vi "Host main_old.vi"() -> ()   [LabVIEW 2013]
uses:
  <vilib>/rvi/interface/nirviReadWriteControl/nirviReadWriteControl.xnode
  <vilib>/rvi/errors/niLvFpgaAdjustHostInterfaceError.vi
  <vilib>/rvi/interface/nirviCloseFPGA/nirviCloseFPGA.xnode
  FPGA/DataMode.ctl
  <vilib>/Utility/error.llb/Error Cluster From Error Code.vi
  <vilib>/rvi/interface/Simulation/niFpgaSimulationCallBeginRW.vi
  Host/Utilities/Ticker/Ticker.lvclass
  Host/Scope/controls/ScopeMode.ctl
  <vilib>/rvi/interface/nirviOpenFPGA/nirviOpenFPGA.xnode
  Host/Scope/P2P streaming/trigger_source.ctl
  Host/Config/FPGAref.ctl
  <userlib>/_OpenG.lib/file/file.llb/Valid Path - Traditional__ogtk.vi
  NiFpgaLv.dll
  FPGA Bitfiles/mixer_FPGATarget_FPGAmain_-FFnNgPrUUY.lvbitx
  <vilib>/FPGAPlugInAG/PXIe-7975R/niLvFpga_Open_PXIe-7975R.vi
  <vilib>/rvi/interface/common/dynamic/niFpgaDynamicAddResources.vi
  <vilib>/FPGAPlugInAG/Dynamic/niLvFpga_Close_Dynamic.vi
  <vilib>/userdefined/High Color/nirio_resource_hc.ctl
  <vilib>/Analysis/4window.llb/windowTd.ctl
  <vilib>/Analysis/NI_AALPro.lvlib
  Host/Scope/controls/power_spectrum_unit.ctl
panel:
  in  "Filter coefficients":path
  in  "Extra downsample":u16(ring) items=["None", "2", "3", "4", "5", "6", "7", "8", "9", "10", "11", "12", "13", "14", "15", "16"]
  in  "Enable extra FIR filter":bool
  in  "Ch1 Q":bool
  in  "Ch1 I":bool
  in  "Ch0 Q":bool
  in  "Ch0 I":bool
  in  "Ch1":bool
  in  "Ch0":bool
  out "stop 2":bool
  out "error out":errorcluster
  in  "Trigger":T1
  in  "Zoom freq X":bool
  in  "Zoom freq Y":bool
  in  "Zoom time Y":bool
  in  "Zoom time X":bool
  in  "Ch3":bool
  in  "Ch2":bool
  in  "Ch3 Q":bool
  in  "Ch3 I":bool
  in  "Ch2 Q":bool
  in  "Ch2 I":bool
  in  "input impedance":u32(ring) caption="Input Impedance" items=["1 mega ohm"=0, "50 ohms"=2]
  in  "SCOPE Resource":refnum<k15>="Dev1" caption="NI-Scope Resource"
  in  "Unit":T2
  in  "Window":T3=1 items=["Rectangle"=0, "Hanning"=1, "Hamming"=2, "Blackman-Harris"=3, "Exact Blackman"=4, "Blackman"=5, "Flat Top"=6, "4 Term B-Harris "=7, "7 Term B-Harris"=8, "Low Sidelobe"=9, "Blackman Nuttall"=11, "Triangle"=30, "Bartlett-Hanning"=31, "Bohman"=32, "Parzen"=33, "Welch"=34, "Kaiser"=60, "Dolph-Chebyshev"=61, "Gaussian"=62]
  in  "Samples per record":u32
  in  "Phase offset (deg)":dbl
  in  "Fequency [MHz]":dbl
  in  "Mode":T4
  in  "Mixer freq [MHz]":dbl
  in  "Ch1":bool
  in  "Ch0":bool
  out "freqdata":cluster{"f0":dbl, "df":dbl, "magnitude":dbl[]}[](graph)
  out "Timedata":i16[][](graph)
  in  "Rumode":bool
  in  "Singleshot":bool
  in  "Ch1 Q":bool
  in  "Ch1 I":bool
  in  "Ch0 Q":bool
  in  "Ch0 I":bool
  out "error IO":errorcluster
  in  "stop":bool
  in  "resource name":T5="RIO0"
  out "Clocking Option Configured?":bool
  out "Configured?":bool
  # "FPGA setup"
  # "Auto Zoom"
  # "Simulated data"
  # "5772"
  # "5160"
  # "Auto Zoom"
  # "FFT"
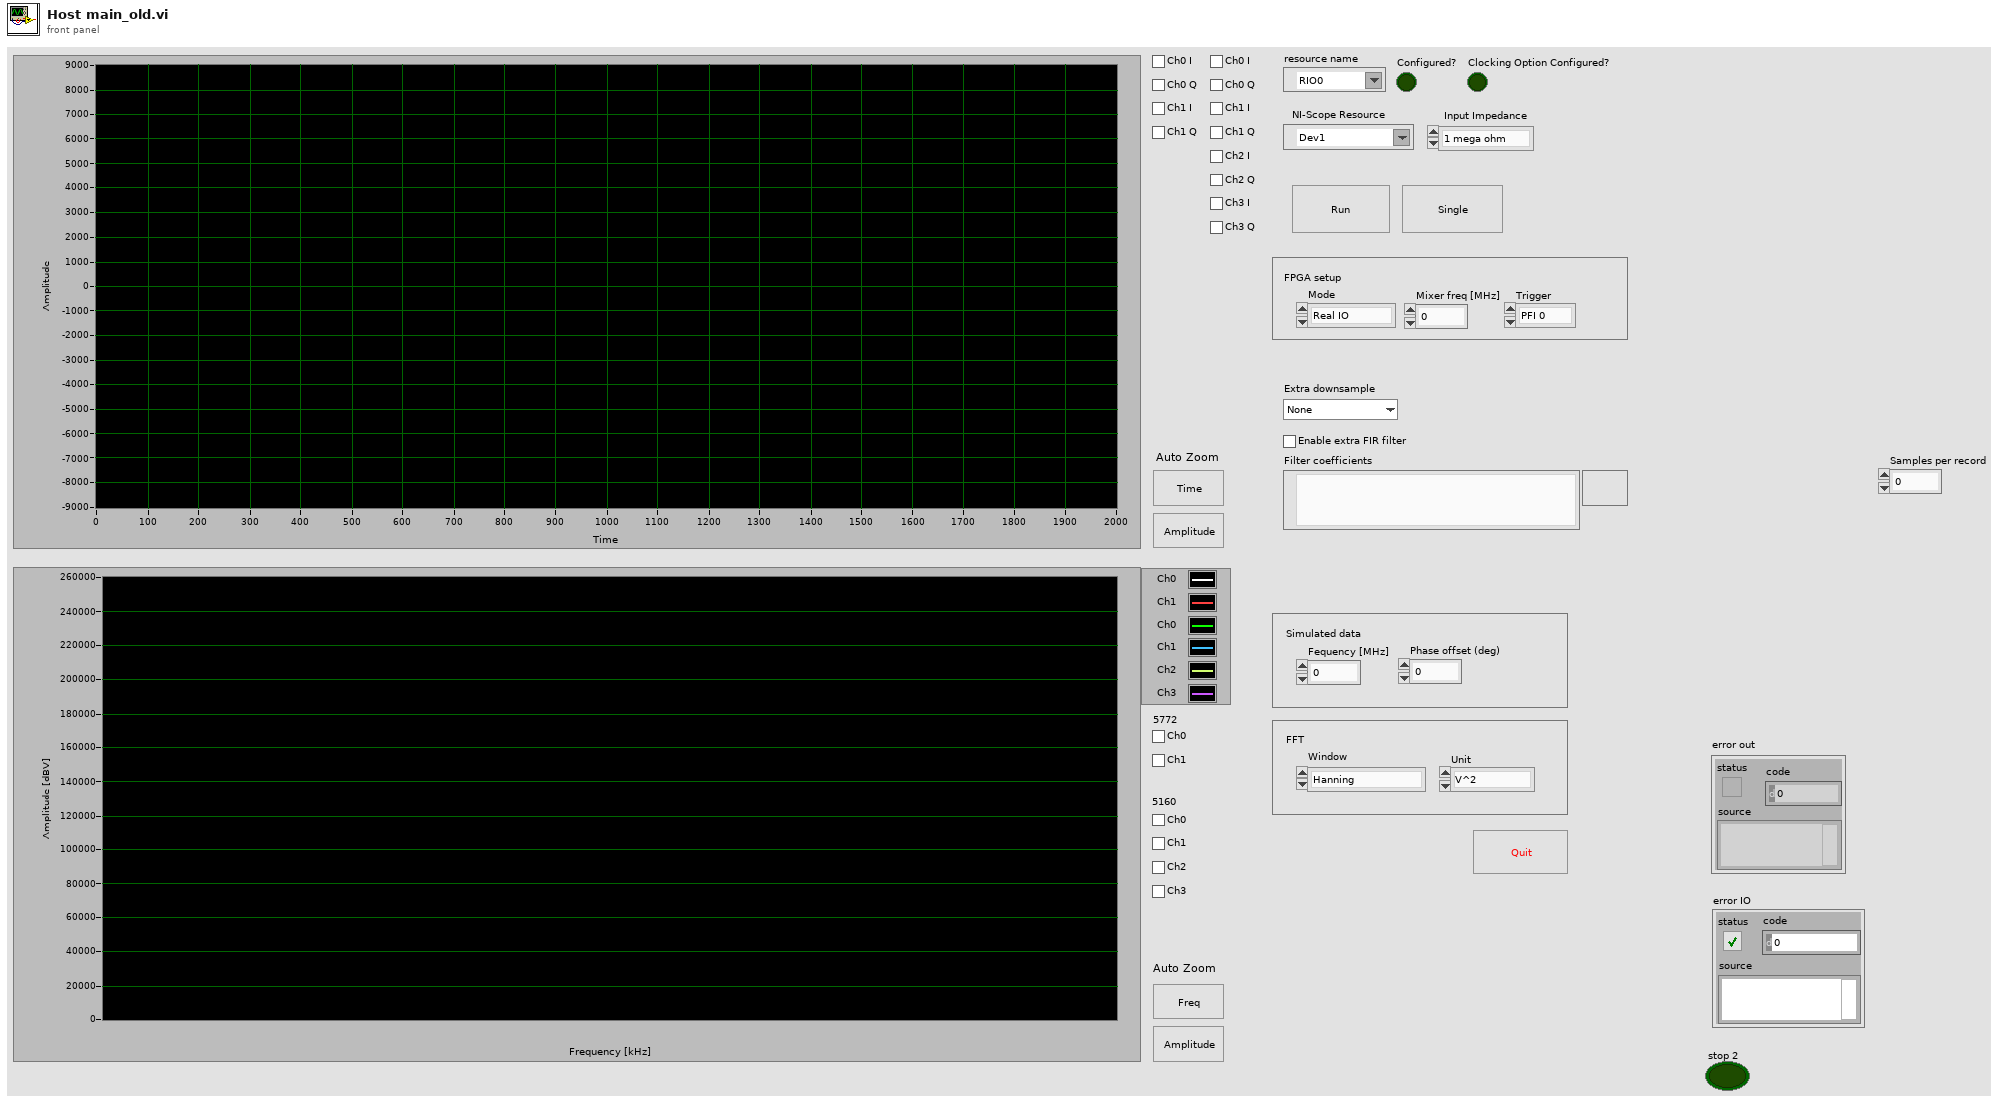
[diagram p1: front panel]
types:
  T1 = typedef "trigger_source.ctl" = enum16{"PFI 0", "PFI 1", "Software"}
  T2 = typedef "power_spectrum_unit.ctl" = enum16{"V^2", "V", "dBV"}
  T3 = typedef "NI_AALPro.lvlib/windowTd.ctl" = u32
  T4 = typedef "DataMode.ctl" = enum16{"Real IO", "Simulated"}
  T5 = typedef "nirio_resource_hc.ctl" = tag
  T6 = enum8{"Internal Clock PLL Off", "Internal Clock PLL On (REF IN)", "External Clock (CLK_IN)", "Internal Clock PLL On (IoModSyncClk)"}
  T7 = typedef "FPGAref.ctl" = refnum<k20>
  T8 = typedef "scope_params.ctl" = cluster{"scope mode":T9, "ticker":refnum<class "Ticker.lvclass">, "5160 samples per trigger":u32, "FPGA ref":T7, "P2P params":T10, "data mode":T4, "5782 samples per record":u32, "Chart length":i32}
  T9 = typedef "ScopeMode.ctl" = enum16{"Stopped", "Single", "Running", "Continuous"}
  T10 = typedef "P2P params.ctl" = cluster{"instrument handle":refnum<k15>, "stream session":refnum<k20>, "scale":cluster{"offset":dbl, "gain":dbl, "reserved 1":dbl, "reserved 2":dbl}, "actual sample rate":dbl, "Trigger":T1, "SCOPE Resource":refnum<k15>, "input impedance":u32}
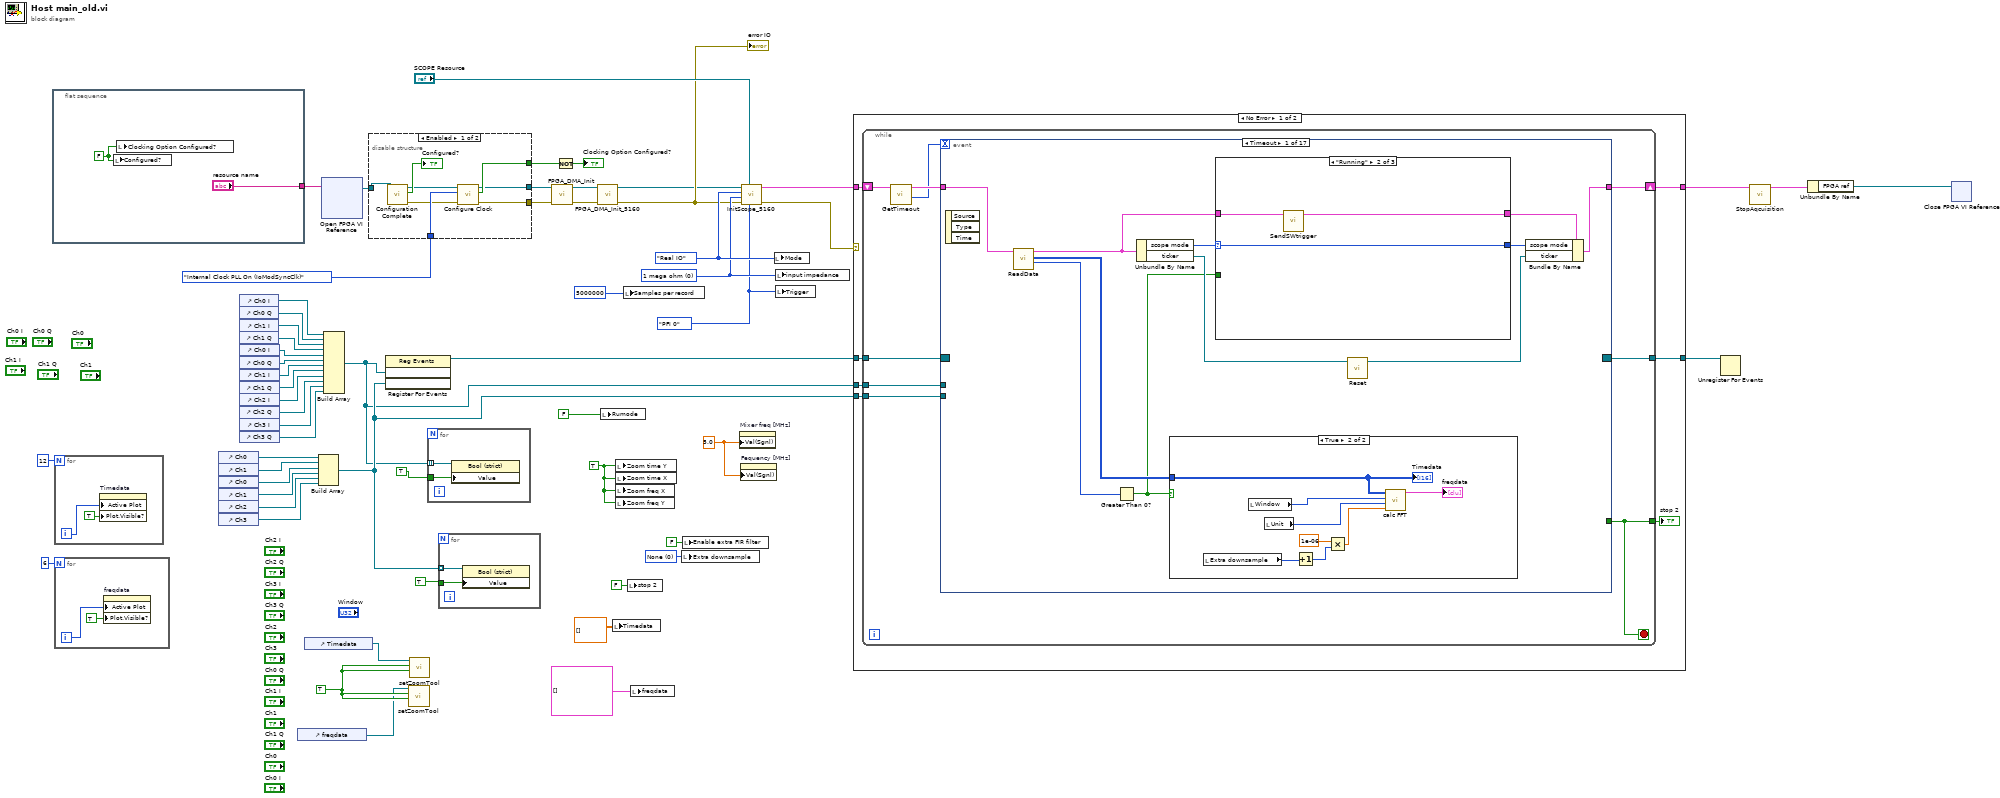
[diagram p0: block diagram]
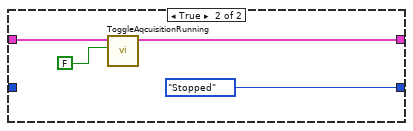
[diagram p6: hidden frame]
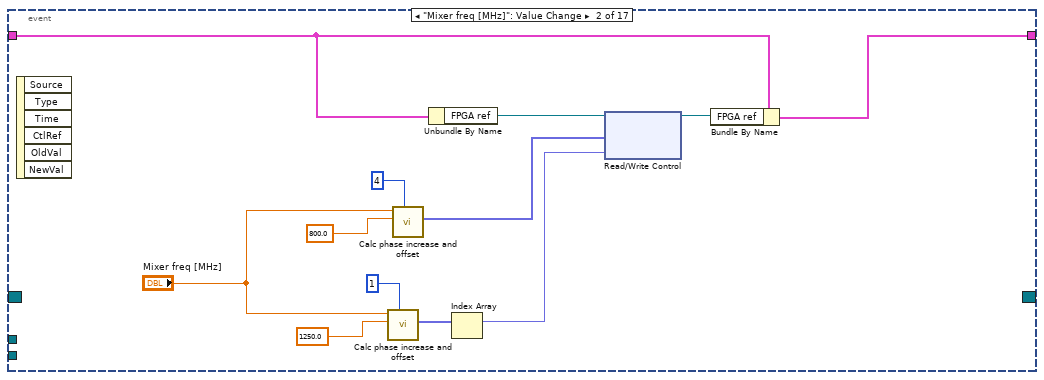
[diagram p7: hidden frame]
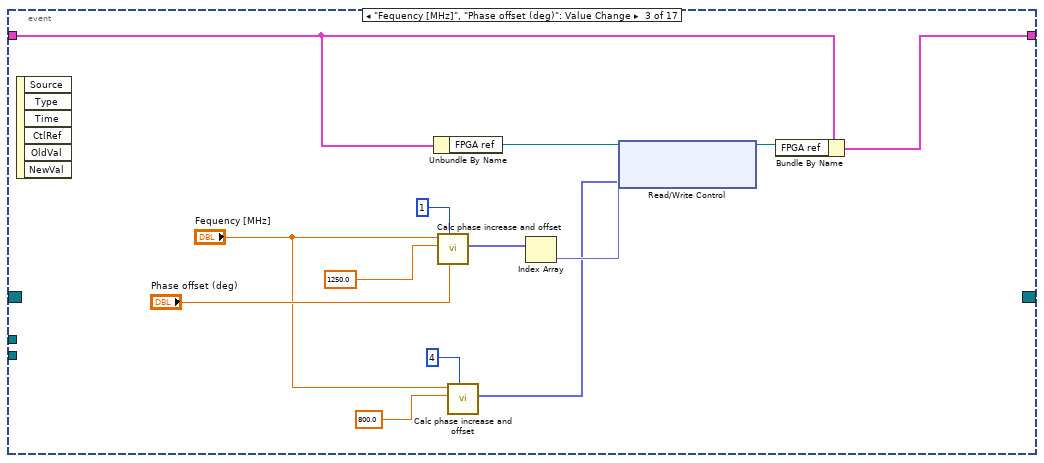
[diagram p8: hidden frame]
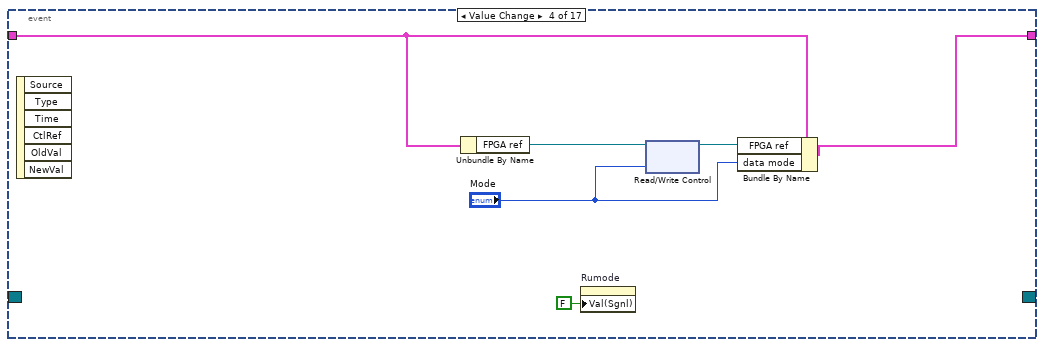
[diagram p9: hidden frame]
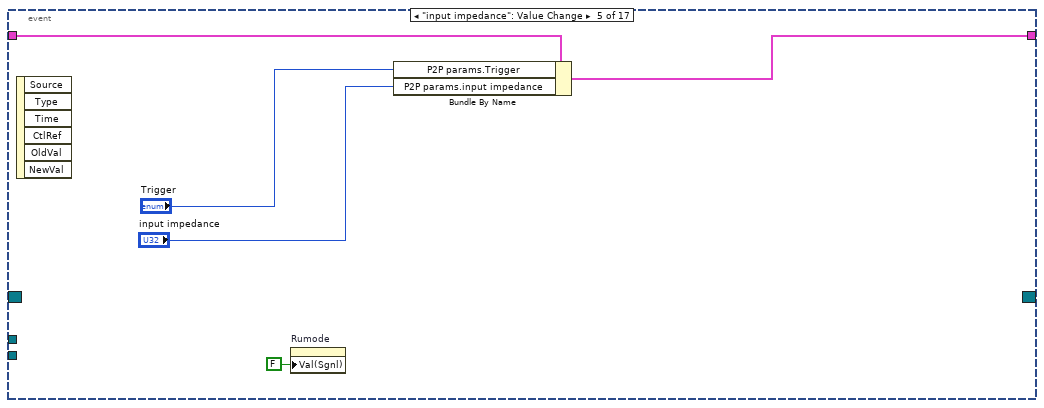
[diagram p10: hidden frame]
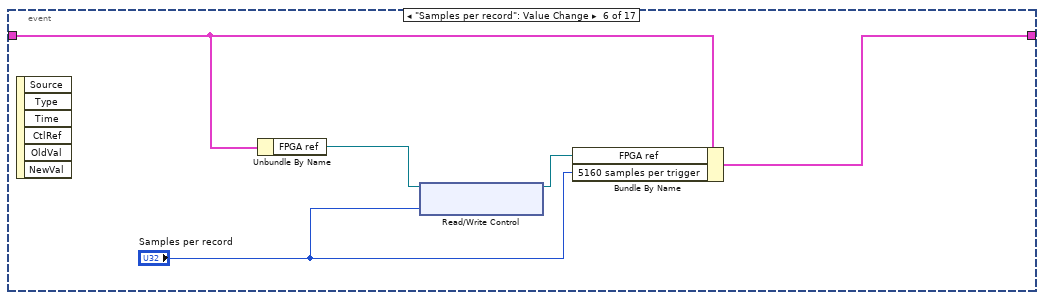
[diagram p11: hidden frame]
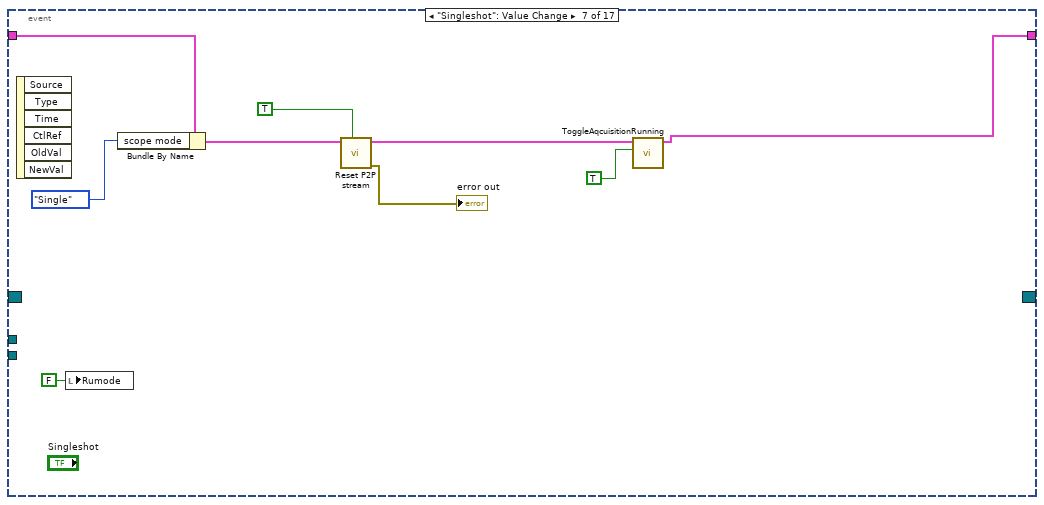
[diagram p12: hidden frame]
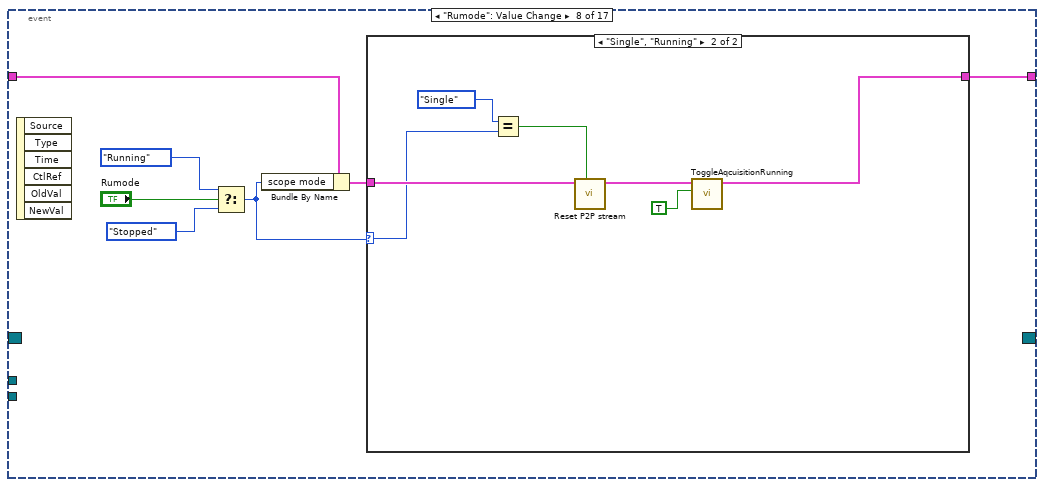
[diagram p13: hidden frame]
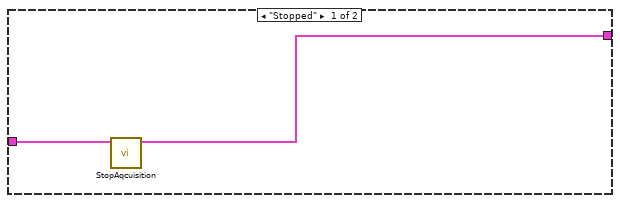
[diagram p14: hidden frame]
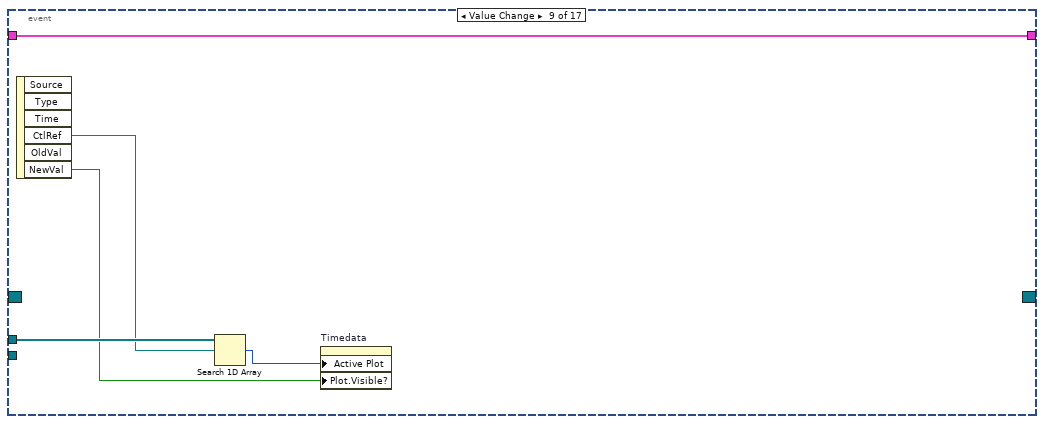
[diagram p15: hidden frame]
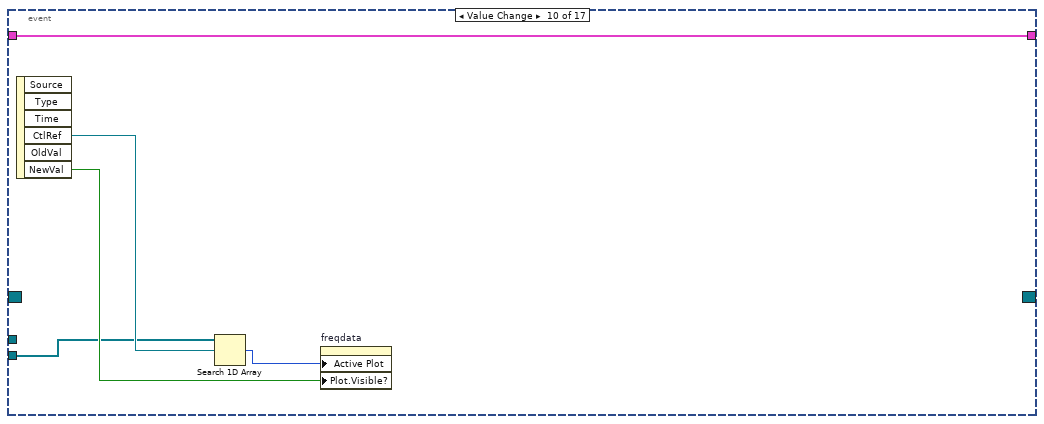
[diagram p16: hidden frame]
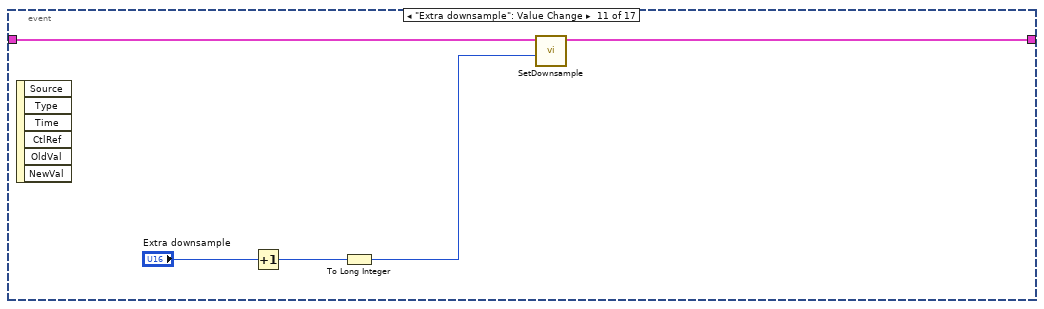
[diagram p17: hidden frame]
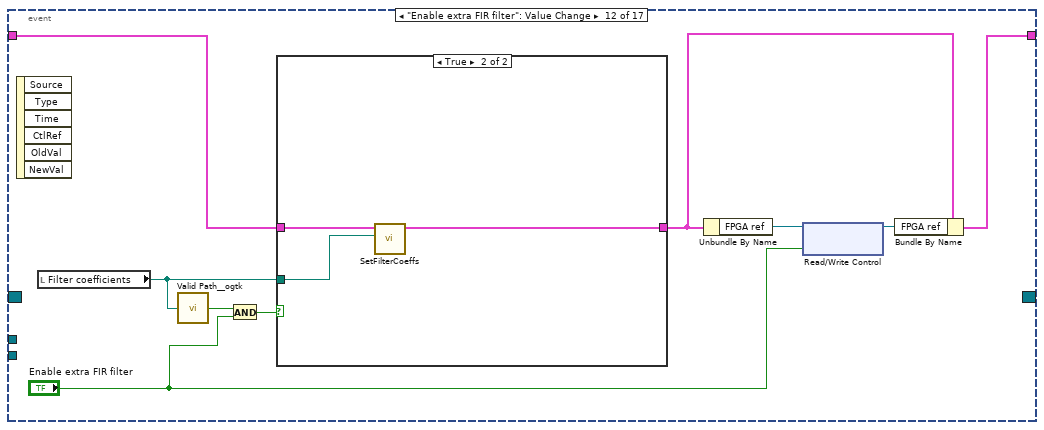
[diagram p18: hidden frame]
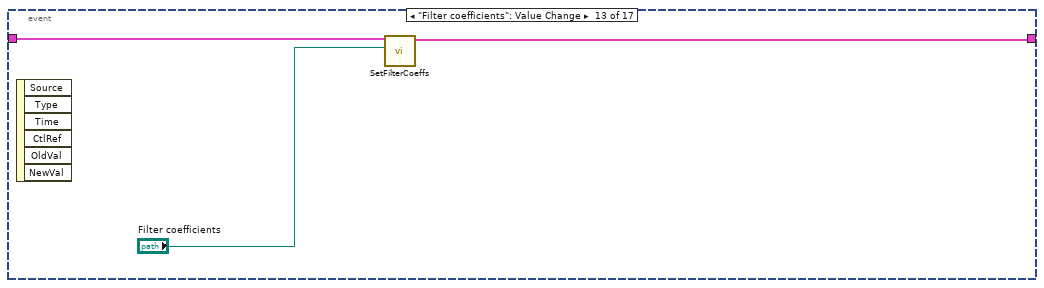
[diagram p20: hidden frame]
diagram:
  w3 = TRUE ("Zoom  X")
  w6 = u16 0 items=["None", "2", "3", "4", "5", "6", "7", "8", "9", "10", "11", "12", "13", "14", "15", "16"] ("Extra downsample")
  w20 = u32 0 items=["1 mega ohm"=0, "50 ohms"=2] ("input impedance")
  w16 = trigger_source."PFI 0" ("Trigger")
  w28 = TRUE ("Rumode")
  w21 = DataMode."Real IO" ("Mode")
  w54 = 5.0 ("Mixer requency [MHz]")
  n1 = flat-sequence {
    tunnel: ["resource name"] -> w29
    frame #0 {
      w59 = FALSE ("Trigger Acquisition")
      n2 = local write "Configured?"(w59) -> ()
      n3 = local write "Clocking Option Configured?"(w59) -> ()
    }
  }
  n4 = for {
    N: 12 -> [_]
    i -> [w62]
    n5 = property on="Timedata" class="WFGraph (strict)"("Active Plot"=w62, "Plot.Visible?"=TRUE ("Plot.Visible")) -> ()  [unwired: 2 in, 2 out]
  }
  n6 = for {
    N: 6 -> [_]
    i -> [w63]
    n7 = property on="freqdata" class="WFGraph (strict)"("Active Plot"=w63, "Plot.Visible?"=TRUE ("Plot.Visible")) -> ()  [unwired: 2 in, 2 out]
  }
  n8 = control-ref of="Ch0"() -> (w11:refnum<vi>)
  n9 = control-ref of="Ch1"() -> (w12:refnum<vi>)
  n10 = control-ref of="Ch0"() -> (w39:refnum<vi>)
  n11 = control-ref of="Ch1"() -> (w38:refnum<vi>)
  n12 = control-ref of="Ch2"() -> (w37:refnum<vi>)
  n13 = control-ref of="Ch3"() -> (w36:refnum<vi>)
  n14 = control-ref of="Ch0 I"() -> (w7:refnum<vi>)
  n15 = control-ref of="Ch0 Q"() -> (w8:refnum<vi>)
  n16 = control-ref of="Ch1 I"() -> (w9:refnum<vi>)
  n17 = control-ref of="Ch1 Q"() -> (w10:refnum<vi>)
  n18 = control-ref of="Ch0 I"() -> (w50:refnum<vi>)
  n19 = control-ref of="Ch0 Q"() -> (w49:refnum<vi>)
  n20 = control-ref of="Ch1 I"() -> (w48:refnum<vi>)
  n21 = control-ref of="Ch1 Q"() -> (w47:refnum<vi>)
  n22 = control-ref of="Ch2 I"() -> (w46:refnum<vi>)
  n23 = control-ref of="Ch2 Q"() -> (w45:refnum<vi>)
  n24 = control-ref of="Ch3 I"() -> (w44:refnum<vi>)
  n25 = control-ref of="Ch3 Q"() -> (w43:refnum<vi>)
  n26 = control-ref of="freqdata"() -> (w1:refnum<vi>)
  n27 = control-ref of="Timedata"() -> (w2:refnum<vi>)
  n28 = Build Array(w11, w12, w39, w38, w37, w36) -> (w34:refnum<vi>[])
  n29 = xnode "Open FPGA VI Reference"("resource name"=w29) -> ("FPGA VI Reference Out"=w26:refnum<k20>)  [unwired: 1 in, 1 out]
  n30 = Build Array(w7, w8, w9, w10, w50, w49, w48, w47, w46, w45, w44, w43) -> (w4:refnum<vi>[])
  n31 = disable-structure shown="Enabled" {
    disable-tunnel: [w71 _] -> w32
    disable-tunnel: T6."Internal Clock PLL On (IoModSyncClk)" ("Clock Source") -> [w70 _]
    disable-tunnel: [w68 _] -> w30
    disable-tunnel: [w67 w73] -> w27
    disable-tunnel: w26 -> [w66 w73]
    frame Enabled {
      n32 = call "Configuration Complete.vi"("FPGA VI Reference in"=w66) -> ("error out"=w69:errorcluster, "Configured?"=→"Configured?":bool, "FPGA VI Reference Out"=w65:T7)  [unwired: 8 in]
      n33 = call "Configure Clock.vi"("error in"=w69, "Clock Source"=w70, "FPGA VI Reference in"=w65) -> ("error out"=w68:errorcluster, "Configuration Error"=w71:bool, "FPGA VI Reference Out"=w67:T7)  [unwired: 6 in]
    }
    frame Disabled {
    }
  }
  n34 = register-events(w4, w34) -> (reference out=w42:refnum<event-registration>)  [unwired: 2 in, 1 out]
  n35 = call "setZoomTool.vi"("Zoom Y"=w3, "Zoom  X"=w3, "reference"=w1) -> ()  [unwired: 9 in]
  n36 = call "setZoomTool.vi"("Zoom Y"=w3, "Zoom  X"=w3, "reference"=w2) -> ()  [unwired: 9 in]
  n37 = for {
    tunnel: w4 -> [w75] mode=indexing
    tunnel: TRUE ("Rumode") -> [w74]
    n38 = property class="Bool (strict)"(reference=w75, "Value"=w74) -> ()  [unwired: 1 in, 2 out]
  }
  n39 = for {
    tunnel: w34 -> [w77] mode=indexing
    tunnel: TRUE ("Rumode") -> [w76]
    n40 = property class="Bool (strict)"(reference=w77, "Value"=w76) -> ()  [unwired: 1 in, 2 out]
  }
  n41 = call "FPGA_DMA_Init.vi"("error in (no error)"=w30, "FPGA VI Reference"=w27) -> ("error out"=w17:errorcluster, "FPGA VI out"=w18:T7)  [unwired: 7 in, 1 out]
  n42 = Not(x=w32) -> (.not. x?=→"Clocking Option Configured?":bool)
  n43 = call "FPGA_DMA_Init_5160.vi"("error in (no error)"=w17, "FPGA VI Reference"=w18) -> ("error out"=w15:errorcluster, "FPGA VI Reference out"=w13:T7)  [unwired: 7 in, 1 out]
  "error IO" <- w15
  n44 = local write "Rumode"(FALSE ("Rumode")) -> ()
  n45 = local write "Timedata"(dbl[][] [] ("Timedata")) -> ()
  n46 = local write "Zoom time Y"(w28) -> ()
  n47 = local write "Zoom time X"(w28) -> ()
  n48 = local write "Zoom freq X"(w28) -> ()
  n49 = local write "Zoom freq Y"(w28) -> ()
  n50 = local write "Samples per record"(u32 5000000 ("Samples to aqcuire")) -> ()
  n51 = local write "stop 2"(FALSE ("stop 2")) -> ()
  n52 = local write "freqdata"(cluster{"f0":dbl, "df":dbl, "magnitude":dbl[]}[] [] ("freqdata")) -> ()
  n53 = local write "Extra downsample"(w6) -> ()
  n54 = local write "Enable extra FIR filter"(FALSE ("Enable extra FIR filter")) -> ()
  n55 = property on="Mixer freq [MHz]" class="DigNum (strict)"("Val(Sgnl)"=w54) -> ()  [unwired: 2 in, 2 out]
  n56 = property on="Fequency [MHz]" class="DigNum (strict)"("Val(Sgnl)"=w54) -> ()  [unwired: 2 in, 2 out]
  n57 = call "InitScope_5160.vi"("Trigger ource"=w16, "SCOPE Resource"="SCOPE Resource", "error in"=w15, "input impedance"=w20, "data mode"=w21, "FPGA ref"=w13) -> ("error out"=w14:errorcluster, "scope params"=w58:T8)  [unwired: 4 in]
  n58 = local write "Mode"(w21) -> ()
  n59 = local write "input impedance"(w20) -> ()
  n60 = local write "Trigger"(w16) -> ()
  n61 = case shown="No Error" w14 {
    tunnel: w58 -> [w84 w246]
    tunnel: [w83 w246] -> w25
    tunnel: w42 -> [w82 w245]
    tunnel: [w81 w245] -> w41
    tunnel: w4 -> [w80 _]
    tunnel: w34 -> [w79 _]
    frame No Error {
      n62 = while {
        shift-right: [w93] -> w83
        shift-left: w84 -> [w92]
        tunnel: w82 -> [w89]
        tunnel: [w88] -> w81
        tunnel: w80 -> [w87]
        tunnel: w79 -> [w86]
        tunnel: [w85] -> w78
        stop <- w85 stop-if-true
        n63 = call "GetTimeout.vi"("scope in"=w92) -> ("Time left"=w90:i32, "scope out"=w91:T8)  [unwired: 9 in]
        n64 = event shown="[0] Timeout" {
          selector: w89 -> [_ _ _ _ _ _ _ _ _ _ _ _ _ _ _ _ _]
          dyn-events: [_ _ _ _ _ _ _ _ _ _ _ _ _ _ _ _ _] -> w88
          timeout: w90 -> [_ _ _ _ _ _ _ _ _ _ _ _ _ _ _ _ _]
          tunnel: [_ _ _ _ _ _ _ _ _ _ _ _ _ "stop" _ _ _] -> w85
          tunnel: w91 -> [w99 w136 w149 w157 w163 w166 w176 w181 w199 w204 w208 w211 w225 w226 w233 w240 w244]
          tunnel: [w102 w134 w148 w156 w160 w165 w170 w179 w199 w204 w207 w216 w224 w226 w233 w240 w244] -> w93
          tunnel: w87 -> [_ _ _ _ _ _ _ _ w198 _ _ _ _ _ _ _ _]
          tunnel: w86 -> [_ _ _ _ _ _ _ _ _ w200 _ _ _ _ _ _ _]
          event Timeout {
            n65 = event-data() -> ()  [unwired: 1 in, 3 out]
            n66 = call "ReadData.vi"("scope params"=w99) -> ("Num elements"=w96:i32, "data"=w95:i16[][], "scope params out"=w98:T8)  [unwired: 8 in]
            n67 = Greater Than 0?(x=w96) -> (x > 0?=w94:bool)
            n68 = Unbundle By Name(w98) -> ("scope mode"=w101:T9, "ticker"=w104:refnum<class "Ticker.lvclass">)
            n69 = case shown="True" w94 {
              tunnel: w95 -> [_ w109]
              frame False {
              }
              frame True {
                n70 = local read "Extra downsample"() -> (w108:u16)
                n71 = local read "Window"() -> (w111:T3)
                n72 = local read "Unit"() -> (w110:T2)
                n73 = Increment(x=w108) -> (x+1=w107:u16)
                n74 = Multiply(x=1e-06 ("dt"), y=w107) -> (x*y=w105:dbl)
                n75 = call "calc FFT.vi"("dt"=w105, "Unit"=w110, "Window"=w111, "data"=w109) -> ("Power Spectrum / PSD"=→"freqdata":cluster{"f0":dbl, "df":dbl, "magnitude":dbl[]}[])  [unwired: 7 in]
                "Timedata" <- w109
              }
            }
            n76 = case shown="\"Running\"" w101 {
              selector: w101 -> [w114 w117 w118]
              tunnel: [w114 w117 w122] -> w100
              tunnel: w98 -> [w113 w116 w121]
              tunnel: [w113 w115 w120] -> w97
              tunnel: w94 -> [_ _ w119]
              frame "Stopped" {
              }
              frame "Running" {
                n77 = call "SendSWtrigger.vi"("scope in"=w116) -> ("scope out"=w115:T8)  [unwired: 9 in, 1 out]
              }
              frame "Single" {
                n78 = case shown="False" w119 {
                  tunnel: [w123 ScopeMode."Stopped" ("scope mode")] -> w122
                  tunnel: w121 -> [w124 w127]
                  tunnel: [w124 w125] -> w120
                  tunnel: w118 -> [w123 _]
                  frame False {
                  }
                  frame True {
                    n79 = call "ToggleAqcuisitionRunning.vi"("Acquisition running"=FALSE, "scope in"=w127) -> ("scope out"=w125:T8)  [unwired: 8 in, 1 out]
                  }
                }
              }
            }
            n80 = call "Reset.vi"("Ticker in"=w104) -> ("Ticker out"=w103:refnum<class "Ticker.lvclass">)  [unwired: 9 in, 1 out]
            n81 = Bundle By Name(cluster=w97, "scope mode"=w100, "ticker"=w103) -> (w102:T8)
          }
          event "Mixer freq [MHz]": Value Change {
            n82 = event-data() -> ()  [unwired: 1 in, 6 out]
            n83 = call "Calc phase increase and offset.vi"("# of DDS"=1, "fclk (MHz)"=1250.0 ("fclk (800MHz)"), "f_generated (MHz)"="Mixer freq [MHz]") -> ("Phase out"=w138:fxp<+,64,64>[])  [unwired: 6 in, 2 out]
            n84 = call "Calc phase increase and offset.vi"("# of DDS"=4, "fclk (MHz)"=800.0 ("fclk (800MHz)"), "f_generated (MHz)"="Mixer freq [MHz]") -> ("Phase out"=w129:fxp<+,64,64>[])  [unwired: 6 in, 2 out]
            n85 = Unbundle By Name(w136) -> ("FPGA ref"=w137:T7)
            n86 = Index Array(array=w138) -> (element=w133:fxp<+,64,64>)  [unwired: 1 in]
            n87 = xnode "Read/Write Control"("FPGA VI Reference In"=w137, "Phase 5772"=w129, "phase 5160"=w133) -> ("FPGA VI Reference Out"=w135:T7)  [unwired: 1 in, 1 out]
            n88 = Bundle By Name(cluster=w136, "FPGA ref"=w135) -> (w134:T8)
          }
          event "Fequency [MHz]", "Phase offset (deg)": Value Change {
            n89 = event-data() -> ()  [unwired: 1 in, 6 out]
            n90 = Unbundle By Name(w149) -> ("FPGA ref"=w151:T7)
            n91 = call "Calc phase increase and offset.vi"("Phase offset (deg)"="Phase offset (deg)", "# of DDS"=1, "fclk (MHz)"=1250.0 ("fclk (800MHz)"), "f_generated (MHz)"="Fequency [MHz]") -> ("Phase out"=w147:fxp<+,64,64>[])  [unwired: 5 in, 2 out]
            n92 = call "Calc phase increase and offset.vi"("# of DDS"=4, "fclk (MHz)"=800.0 ("fclk (800MHz)"), "f_generated (MHz)"="Fequency [MHz]") -> ("Phase out"=w141:fxp<+,64,64>[])  [unwired: 6 in, 2 out]
            n93 = Index Array(array=w147) -> (element=w145:fxp<+,64,64>)  [unwired: 1 in]
            n94 = xnode "Read/Write Control"("FPGA VI Reference In"=w151, "simulated phase 51600"=w145, "Simulated phase 5772"=w141) -> ("FPGA VI Reference Out"=w150:T7)  [unwired: 1 in, 1 out]
            n95 = Bundle By Name(cluster=w149, "FPGA ref"=w150) -> (w148:T8)
          }
          event Value Change {
            n96 = event-data() -> ()  [unwired: 1 in, 6 out]
            n97 = Unbundle By Name(w157) -> ("FPGA ref"=w159:T7)
            n98 = property on="Rumode" class="Bool (strict)"("Val(Sgnl)"=FALSE ("Value (Signaling)")) -> ()  [unwired: 2 in, 2 out]
            n99 = xnode "Read/Write Control"("FPGA VI Reference In"=w159, "Mode"="Mode") -> ("FPGA VI Reference Out"=w158:T7)  [unwired: 1 in, 1 out]
            n100 = Bundle By Name(cluster=w157, "FPGA ref"=w158, "data mode"="Mode") -> (w156:T8)
          }
          event "input impedance": Value Change {
            n101 = event-data() -> ()  [unwired: 1 in, 6 out]
            n102 = property on="Rumode" class="Bool (strict)"("Val(Sgnl)"=FALSE ("Value (Signaling)")) -> ()  [unwired: 2 in, 2 out]
            n103 = Bundle By Name(cluster=w163, "P2P params.Trigger"="Trigger", "P2P params.input impedance"="input impedance") -> (w160:T8)
          }
          event "Samples per record": Value Change {
            n104 = event-data() -> ()  [unwired: 1 in, 6 out]
            n105 = Unbundle By Name(w166) -> ("FPGA ref"=w169:T7)
            n106 = xnode "Read/Write Control"("FPGA VI Reference In"=w169, "Samples Per Trigger"="Samples per record") -> ("FPGA VI Reference Out"=w168:T7)  [unwired: 1 in, 1 out]
            n107 = Bundle By Name(cluster=w166, "FPGA ref"=w168, "5160 samples per trigger"="Samples per record") -> (w165:T8)
          }
          event "Singleshot": Value Change {
            n108 = event-data() -> ()  [unwired: 1 in, 6 out]
            n109 = local write "Rumode"(FALSE ("Rumode")) -> ()
            n110 = Bundle By Name(cluster=w176, "scope mode"=ScopeMode."Single") -> (w175:T8)
            n111 = call "Reset P2P stream.vi"("single shot"=TRUE, "scope params"=w175) -> ("error out"=→"error out":errorcluster, "scope params out"=w171:T8)  [unwired: 8 in]
            n112 = call "ToggleAqcuisitionRunning.vi"("Acquisition running"=TRUE, "scope in"=w171) -> ("scope out"=w170:T8)  [unwired: 8 in, 1 out]
          }
          event "Rumode": Value Change {
            n113 = event-data() -> ()  [unwired: 1 in, 6 out]
            n114 = Select(t=ScopeMode."Running" ("scope mode"), s="Rumode", f=ScopeMode."Stopped" ("scope mode")) -> (s? t:f=w180:T9)
            n115 = Bundle By Name(cluster=w181, "scope mode"=w180) -> (w182:T8)
            n116 = case shown="\"Single\", \"Running\"" w180 {
              selector: w180 -> [_ w190]
              tunnel: w182 -> [w187 w194]
              tunnel: [w186 w192] -> w179
              frame "Stopped" {
                n117 = call "StopAqcuisition.vi"("scope in"=w187) -> ("scope out"=w186:T8)  [unwired: 9 in, 1 out]
              }
              frame "Single", "Running" {
                n118 = Equal?(x=ScopeMode."Single" ("scope mode"), y=w190) -> (x = y?=w188:bool)
                n119 = call "Reset P2P stream.vi"("single shot"=w188, "scope params"=w194) -> ("scope params out"=w193:T8)  [unwired: 8 in, 1 out]
                n120 = call "ToggleAqcuisitionRunning.vi"("Acquisition running"=TRUE, "scope in"=w193) -> ("scope out"=w192:T8)  [unwired: 8 in, 1 out]
              }
            }
          }
          event Value Change {
            n121 = event-data() -> ("CtlRef"=w197:refnum<vi>, "NewVal"=w195:bool)  [unwired: 1 in, 4 out]
            n122 = Search 1D Array(1D array=w198, element=w197) -> (index of element=w196:i32)  [unwired: 1 in]
            n123 = property on="Timedata" class="WFGraph (strict)"("Active Plot"=w196, "Plot.Visible?"=w195) -> ()  [unwired: 2 in, 2 out]
          }
          event Value Change {
            n124 = event-data() -> ("CtlRef"=w203:refnum<vi>, "NewVal"=w201:bool)  [unwired: 1 in, 4 out]
            n125 = Search 1D Array(1D array=w200, element=w203) -> (index of element=w202:i32)  [unwired: 1 in]
            n126 = property on="freqdata" class="WFGraph (strict)"("Active Plot"=w202, "Plot.Visible?"=w201) -> ()  [unwired: 2 in, 2 out]
          }
          event "Extra downsample": Value Change {
            n127 = event-data() -> ()  [unwired: 1 in, 6 out]
            n128 = Increment(x="Extra downsample") -> (x+1=w206:u16)
            n129 = To Long Integer(number=w206) -> (32bit integer=w205:i32)
            n130 = call "SetDownsample.vi"("Downsample rate"=w205, "scope in"=w208) -> ("scope out"=w207:T8)  [unwired: 9 in]
          }
          event "Enable extra FIR filter": Value Change {
            n131 = event-data() -> ()  [unwired: 1 in, 6 out]
            n132 = local read "Filter coefficients"() -> (w212:path)
            n133 = call-poly <userlib>:"Valid Path__ogtk.vi"("path"=w212) -> ("valid"=w215:bool)
            n134 = And(x=w215, y="Enable extra FIR filter") -> (x .and. y?=w213:bool)
            n135 = case shown="True" w213 {
              tunnel: w212 -> [_ w222]
              tunnel: w211 -> [w219 w221]
              tunnel: [w219 w220] -> w210
              frame False {
              }
              frame True {
                n136 = call "SetFilterCoeffs.vi"("COE file"=w222, "scope in"=w221) -> ("scope out"=w220:T8)  [unwired: 8 in, 1 out]
              }
            }
            n137 = Unbundle By Name(w210) -> ("FPGA ref"=w218:T7)
            n138 = xnode "Read/Write Control"("FPGA VI Reference In"=w218, "enable filter"="Enable extra FIR filter") -> ("FPGA VI Reference Out"=w217:T7)  [unwired: 1 in, 1 out]
            n139 = Bundle By Name(cluster=w210, "FPGA ref"=w217) -> (w216:T8)
          }
          event "Filter coefficients": Value Change {
            n140 = event-data() -> ()  [unwired: 1 in, 6 out]
            n141 = call "SetFilterCoeffs.vi"("COE file"="Filter coefficients", "scope in"=w225) -> ("scope out"=w224:T8)  [unwired: 8 in, 1 out]
          }
          event "stop": Value Change {
            n142 = event-data() -> ()  [unwired: 1 in, 6 out]
          }
          event Value Change {
            n143 = event-data() -> ()  [unwired: 1 in, 6 out]
            n144 = case shown="\"V\"" "Unit" {
              tunnel: ["V" "dBV" "V^2"] -> w230
              frame "V" {
              }
              frame "dBV" {
              }
              frame "V^2" {
              }
            }
            n145 = Concatenate Strings("Amplitude [", w230, "]") -> (w228:string)
            n146 = property on="freqdata" class="WFGraph (strict)"("YScale.NameLbl.Text"=w228) -> ()  [unwired: 2 in, 2 out]
          }
          event "Zoom time X", "Zoom time Y": Value Change {
            n147 = event-data() -> ()  [unwired: 1 in, 6 out]
            n148 = control-ref of="Timedata"() -> (w239:refnum<vi>)
            n149 = call "setZoomTool.vi"("Zoom Y"="Zoom time Y", "Zoom  X"="Zoom time X", "reference"=w239) -> ()  [unwired: 9 in]
          }
          event "Zoom freq Y", "Zoom freq X": Value Change {
            n150 = event-data() -> ()  [unwired: 1 in, 6 out]
            n151 = control-ref of="freqdata"() -> (w241:refnum<vi>)
            n152 = call "setZoomTool.vi"("Zoom Y"="Zoom freq Y", "Zoom  X"="Zoom freq X", "reference"=w241) -> ()  [unwired: 9 in]
          }
        }
      }
      "stop 2" <- w78
    }
    frame Error {
    }
  }
  n153 = Unregister For Events(event registration refnum=w41) -> ()  [unwired: 1 in, 1 out]
  n154 = call "StopAqcuisition.vi"("scope in"=w25) -> ("scope out"=w24:T8)  [unwired: 9 in, 1 out]
  n155 = Unbundle By Name(w24) -> ("FPGA ref"=w57:T7)
  n156 = xnode "Close FPGA VI Reference"("FPGA VI Reference In"=w57) -> ()  [unwired: 1 in, 1 out]
